vi "Filter Plugins.vi"(8 "error in (no error)":errorcluster, 10 "Plugin Type":T3, 11 "Full Plugin Array":T1[](array[typedef])) -> (0 "error out":errorcluster, 2 "Filtered Plugin Array out":T1[](array[typedef]), 3 "Full Plugin Array out (dup)":T1[](array[typedef]))   [LabVIEW 2020]
doc: "Filters the list of plugins for only those of the given plugin type."
uses:
  Plugin Manager/Plugin Details.ctl
  Plugin Servers/Controller/Controller Type.ctl
  Plugin Manager/Plugin Types.ctl
  Plugin Manager/Plugin Manager.lvlib
  Plugin Servers/Controller/Generic Plugin.lvclass
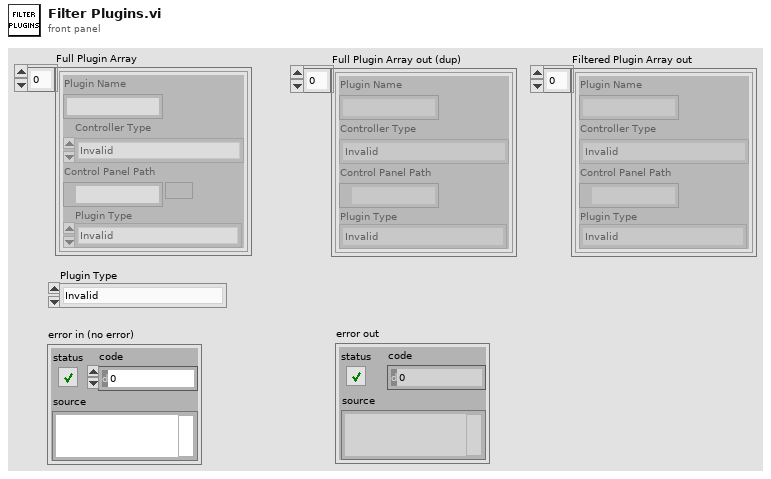
[diagram p1: front panel]
types:
  T1 = typedef "Plugin Manager.lvlib/Plugin Details.ctl" = cluster{"Plugin Name":string, "Controller Type":T2, "Control Panel Path":path, "Plugin Type":T3}
  T2 = typedef "Generic Plugin.lvclass/Controller Type.ctl" = enum16{"Invalid", "Temperature Controller", "Pump Controller", "Generic Optimizer", "LC Parser"}
  T3 = typedef "Plugin Manager.lvlib/Plugin Types.ctl" = enum16{"Invalid", "Optimizer", "Analyzer", "Hardware"}
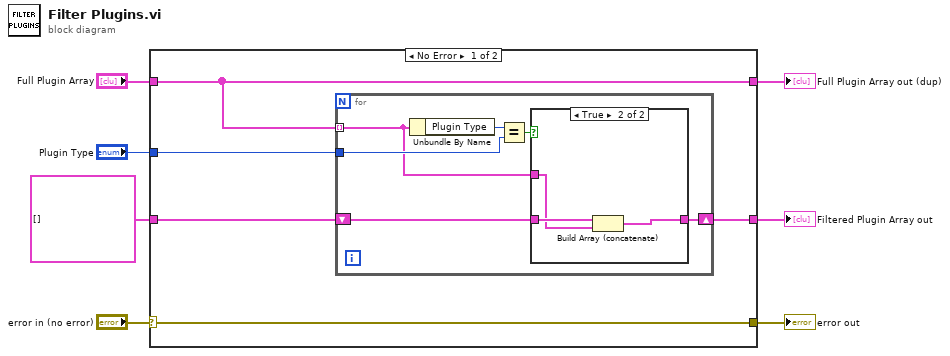
[diagram p0: block diagram]
diagram:
  n1 = case shown="No Error" "error in (no error)" {
    selector: "error in (no error)" -> [w11 w24]
    tunnel: "Plugin Type" -> [w12 _]
    tunnel: "Full Plugin Array" -> [w9 w25]
    tunnel: [w11 w24] -> w4
    tunnel: [w10 w23] -> w3
    tunnel: [w9 w25] -> w2
    tunnel: T1[] [] ("Plugin Array") -> [w8 w23]
    frame No Error {
      n2 = for {
        tunnel: w9 -> [w15] mode=indexing
        tunnel: w12 -> [w17]
        shift-right: [w13] -> w10
        shift-left: w8 -> [w14]
        n3 = Unbundle By Name(w15) -> ("Plugin Type"=w18:T3)
        n4 = Equal?(x=w18, y=w17) -> (x = y?=w16:bool)
        n5 = case shown="True" w16 {
          tunnel: w15 -> [_ w20]
          tunnel: w14 -> [w19 w22]
          tunnel: [w19 w21] -> w13
          frame False {
          }
          frame True {
            n6 = Build Array (concatenate)(w22, w20) -> (w21:T1[])
          }
        }
      }
    }
    frame Error {
    }
  }
  "error out" <- w4
  "Filtered Plugin Array out" <- w3
  "Full Plugin Array out (dup)" <- w2
